vi "Demo para panther Dasboard.vi"   [LabVIEW 2019]
uses:
  Libraries/PowerElectronics0X45/PowerElectronics0X45.lvlib
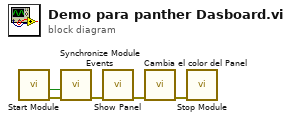
[diagram p0: block diagram]
diagram:
  n1 = call "Start Module.vi"() -> ("error out"=w5:errorcluster, "Wait for Event Sync?"=w4:bool)  [unwired: 7 in, 3 out]
  n2 = call "Synchronize Module Events.vi"("error in"=w5, "Wait for Event Sync?"=w4) -> ("error out"=w3:errorcluster)  [unwired: 9 in]
  n3 = call "Show Panel.vi"("error in"=w3) -> ("error out"=w2:errorcluster)  [unwired: 10 in]
  n4 = call "Cambia el color del Panel.vi"("error in"=w2) -> ("error out"=w1:errorcluster)  [unwired: 10 in]
  n5 = call "Stop Module.vi"("error in"=w1) -> ()  [unwired: 10 in, 1 out]
